vi "Entry.vi"(8 "error in (no error)":errorcluster, 11 "New State":refnum<class "CAncel_Transaction.lvclass">) -> (0 "error out":errorcluster, 3 "State out":refnum<class "CAncel_Transaction.lvclass">)   [LabVIEW 2025, in "ATM_UI_Controller.lvlib" / "CAncel_Transaction.lvclass"]
doc: "This is an abstract method. Override this method to define the behavior when you enter the state."
uses:
  CAncel_Transaction.lvclass
  CAncel_Transaction.lvclass/CAncel_Transaction.ctl
  ATM_UI_Controller.lvclass
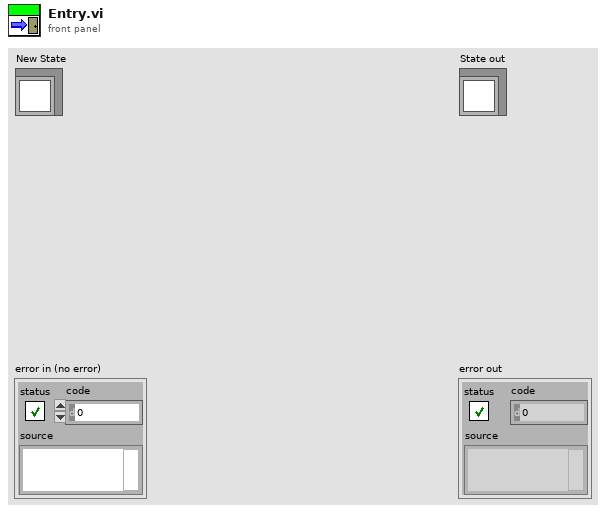
[diagram p1: front panel]
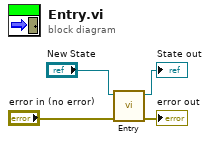
[diagram p0: block diagram]
diagram:
  n1 = call-parent "Entry.vi"("error in (no error)"="error in (no error)", "New State"="New State") -> ("error out"=→"error out":errorcluster, "State out"=→"State out":refnum<class "CAncel_Transaction.lvclass">)  [unwired: 8 in]
